vi "FINALPELLET_Jaredcopy.vi"(0 "NXT/EV3":T1) -> (1 "Material Binary":string, 2 "Type Binary":string)   [LabVIEW 2016]
uses:
  <vilib>/NXT/Subs/LVHSConnector.ctl
  <vilib>/NXT/LegoClasses/BrickReference/BrickReference.lvclass
  <vilib>/NXT/Block Support/NXT_InputPort.ctl
  <vilib>/NXT/Block Support/NXT_OutputPort.ctl
  <vilib>/NXT/Dual Mode Library/Sensors/EV3_Color_Color.vi
  <vilib>/NXT/NXTIO Xnodes/NXTIONodeSubVIs/NXTMotorRunDistance.vi
  <vilib>/NXT/Dual Mode Library/Waits/Wait_Num.vi
  <vilib>/NXT/NXTIO Xnodes/NXTIONodeSubVIs/NXTStopMotors.vi
  <vilib>/NXT/Dual Mode Library/Sensors/EV3_Color_RGB.vi
  <vilib>/NXT/NXTIO Xnodes/AddressXNode/NXTIOAddress.xnode
  <vilib>/NXT/NXTIO Xnodes/NXTIOXNode/NXTIO.xnode
panel:
  out "Material":dbl[](array[numeric])
  out "Type":dbl[](array[numeric])
  in  "Time 2":dbl
  in  "Pause":dbl
  in  "Time 1":dbl
  out "Type":string[](array[string])
  out "Type Binary":string[](array[string])
  out "Material":string[](array[string])
  out "Material Binary":string[](array[string])
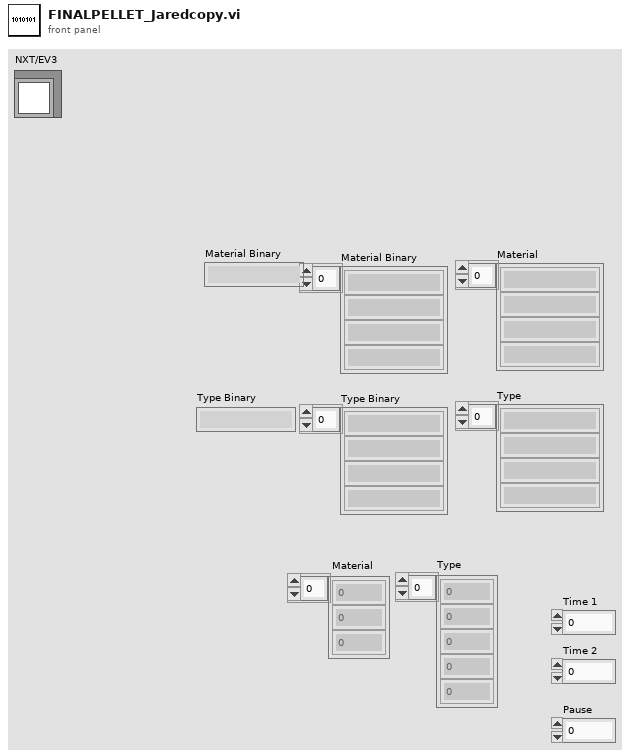
[diagram p1: front panel]
types:
  T1 = typedef "LVHSConnector.ctl" = refnum<class "BrickReference.lvclass">
  T2 = typedef "NXT_InputPort.ctl" = u32
  T3 = typedef "ColorSensorColors.ctl" = enum16{"No Color", "Black", "Blue", "Green", "Yellow", "Red", "White", "Brown"}
  T4 = typedef "NXT_OutputPort.ctl" = u8
  T5 = cluster{"[0]":string, "[1]":string, "[2]":string, "[3]":string, "[4]":string, "[5]":string, "[6]":string, "[7]":string, "[8]":string}
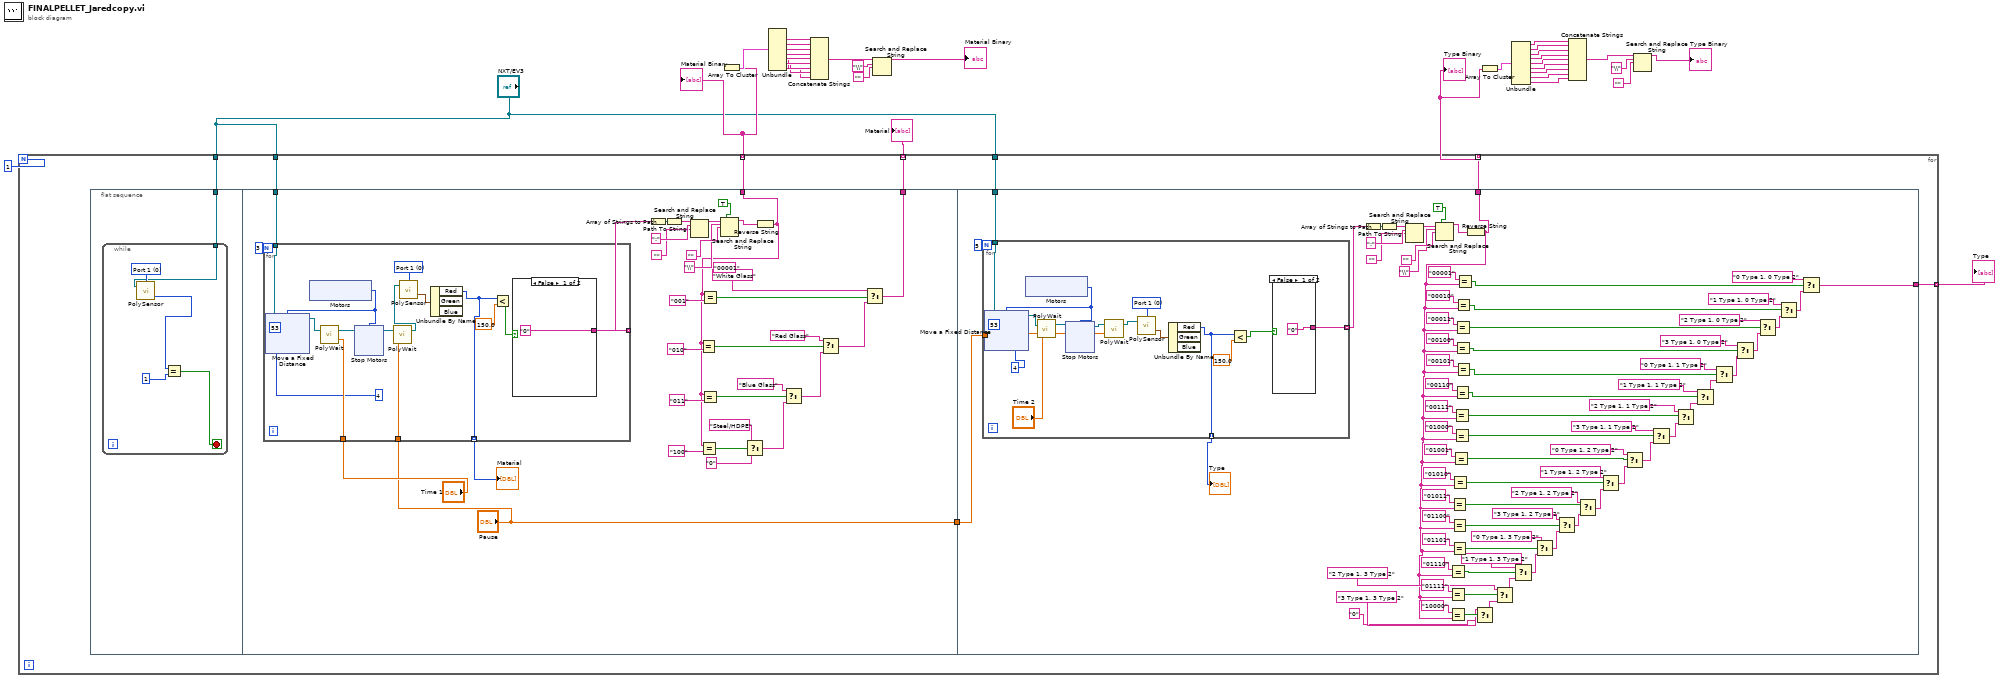
[diagram p0: block diagram]
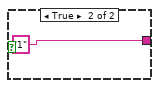
[diagram p2: hidden frame]
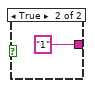
[diagram p3: hidden frame]
diagram:
  n1 = for {
    N: 1 -> [_]
    tunnel: [w42] -> w33 mode=indexing
    tunnel: [w41] -> w32 mode=indexing
    tunnel: [w40] -> w31 mode=indexing
    tunnel: [w39] -> w10 mode=indexing
    tunnel: "NXT/EV3" -> [w37]
    tunnel: "NXT/EV3" -> [w36]
    tunnel: "NXT/EV3" -> [w35]
    n2 = flat-sequence {
      tunnel: w37 -> [w43]
      tunnel: [w66] -> w42
      tunnel: [w52] -> w39
      tunnel: ["Pause"] -> w38
      tunnel: w36 -> [w49]
      tunnel: [w129] -> w41
      tunnel: [w117] -> w40
      tunnel: w38 -> [w121]
      tunnel: w35 -> [w116]
      frame #0 {
        n3 = while {
          tunnel: w43 -> [w44]
          stop <- w46 stop-if-true
          w45 = T2 0 items=["Port 1", "Port 2", "Port 3", "Port 4"] ("Port (Port 1)")
          n4 = call-poly <vilib>:"PolySensor.vi"("NXT/EV3"=w44, "Port (Port 1)"=w45) -> ("Detected Color"=w48:T3)  [unwired: 1 in, 1 out]
          n5 = Equal?(x=w48, y=1) -> (x = y?=w46:bool)
        }
      }
      frame #1 {
        (unwired) "00001"
        n6 = for {
          N: 3 -> [_]
          tunnel: [w97] -> w54 mode=indexing
          tunnel: "Time 1" -> [w95]
          tunnel: "Pause" -> [w93]
          tunnel: [w88] -> w55 mode=indexing
          tunnel: w49 -> [w82]
          w92 = T2 0 items=["Port 1", "Port 2", "Port 3", "Port 4"] ("Port (Port 1)")
          n7 = xnode "Motors"() -> ("Motor"=w84:T4)
          n8 = xnode "Move a Fixed Distance"("Speed 1"=4, "Distance 1"=53, "Motors"=w84, "NXT/EV3"=w82) -> ("NXT/EV3"=w85:T1)
          n9 = call-poly <vilib>:"PolyWait.vi"("Time (1 sec)"=w95, "NXT/EV3"=w85) -> ("NXT/EV3"=w96:T1)  [unwired: 2 in]
          n10 = xnode "Stop Motors"("Motors"=w84, "NXT/EV3"=w96) -> ("NXT/EV3"=w94:T1)
          n11 = call-poly <vilib>:"PolyWait.vi"("Time (1 sec)"=w93, "NXT/EV3"=w94) -> ("NXT/EV3"=w89:T1)  [unwired: 2 in]
          n12 = call-poly <vilib>:"PolySensor.vi"("NXT/EV3"=w89, "Port (Port 1)"=w92) -> ("RGB Color"=w87:cluster{"Red":u8, "Green":u8, "Blue":u8})  [unwired: 1 in, 1 out]
          n13 = Unbundle By Name(w87) -> ("Red"=w88:u8)  [unwired: 2 out]
          n14 = Less?(x=w88, y=150.0) -> (x < y?=w90:bool)
          n15 = case shown="False" w90 {
            tunnel: ["0" "1"] -> w97
            frame False {
            }
            frame True {
            }
          }
        }
        "Material" <- w55
        n16 = Array of Strings to Path(0:w54) -> (2:w65:path)  [unwired: 1 in]
        n17 = Path To String(path=w65) -> (string=w64:string)
        n18 = Search and Replace String(input string=w64, search string=":", replace string="") -> (result string=w61:string)  [unwired: 5 in, 3 out]
        n19 = Search and Replace String(replace all?=TRUE, input string=w61, search string="\\", replace string="") -> (result string=w53:string)  [unwired: 4 in, 3 out]
        n20 = Reverse String(1:w53) -> (0:w52:string)
        n21 = Equal?(x=w52, y="010") -> (x = y?=w51:bool)
        n22 = Equal?(x=w52, y="100") -> (x = y?=w70:bool)
        n23 = Equal?(x=w52, y="011") -> (x = y?=w71:bool)
        n24 = Equal?(x=w52, y="001") -> (x = y?=w50:bool)
        n25 = Select(t="Steel/HDPE", s=w70, f="0") -> (s? t:f=w69:string)
        n26 = Select(t="Blue Glass", s=w71, f=w69) -> (s? t:f=w73:string)
        n27 = Select(t="Red Glass", s=w51, f=w73) -> (s? t:f=w75:string)
        n28 = Select(t="White Glass", s=w50, f=w75) -> (s? t:f=w66:string)
      }
      frame #2 {
        n29 = for {
          N: 5 -> [_]
          tunnel: [w210] -> w119 mode=indexing
          tunnel: w121 -> [w208]
          tunnel: [w201] -> w120 mode=indexing
          tunnel: w116 -> [w196]
          w211 = T2 0 items=["Port 1", "Port 2", "Port 3", "Port 4"] ("Port (Port 1)")
          n30 = xnode "Motors"() -> ("Motor"=w198:T4)
          n31 = xnode "Move a Fixed Distance"("Speed 1"=4, "Distance 1"=53, "Motors"=w198, "NXT/EV3"=w196) -> ("NXT/EV3"=w199:T1)
          n32 = call-poly <vilib>:"PolyWait.vi"("Time (1 sec)"="Time 2", "NXT/EV3"=w199) -> ("NXT/EV3"=w209:T1)  [unwired: 2 in]
          n33 = xnode "Stop Motors"("Motors"=w198, "NXT/EV3"=w209) -> ("NXT/EV3"=w207:T1)
          n34 = call-poly <vilib>:"PolyWait.vi"("Time (1 sec)"=w208, "NXT/EV3"=w207) -> ("NXT/EV3"=w206:T1)  [unwired: 2 in]
          n35 = call-poly <vilib>:"PolySensor.vi"("NXT/EV3"=w206, "Port (Port 1)"=w211) -> ("RGB Color"=w204:cluster{"Red":u8, "Green":u8, "Blue":u8})  [unwired: 1 in, 1 out]
          n36 = Unbundle By Name(w204) -> ("Red"=w201:u8)  [unwired: 2 out]
          n37 = Less?(x=w201, y=150.0) -> (x < y?=w202:bool)
          n38 = case shown="False" w202 {
            tunnel: ["0" "1"] -> w210
            frame False {
            }
            frame True {
            }
          }
        }
        "Type" <- w120
        n39 = Array of Strings to Path(0:w119) -> (2:w194:path)  [unwired: 1 in]
        n40 = Path To String(path=w194) -> (string=w128:string)
        n41 = Search and Replace String(input string=w128, search string=":", replace string="") -> (result string=w125:string)  [unwired: 5 in, 3 out]
        n42 = Search and Replace String(replace all?=TRUE, input string=w125, search string="\\", replace string="") -> (result string=w118:string)  [unwired: 4 in, 3 out]
        n43 = Reverse String(1:w118) -> (0:w117:string)
        n44 = Equal?(x="01111", y=w117) -> (x = y?=w176:bool)
        n45 = Equal?(x="10000", y=w117) -> (x = y?=w177:bool)
        n46 = Equal?(x="01110", y=w117) -> (x = y?=w175:bool)
        n47 = Equal?(x="01011", y=w117) -> (x = y?=w172:bool)
        n48 = Equal?(x="01100", y=w117) -> (x = y?=w173:bool)
        n49 = Equal?(x="01101", y=w117) -> (x = y?=w174:bool)
        n50 = Equal?(x="01010", y=w117) -> (x = y?=w171:bool)
        n51 = Equal?(x="01001", y=w117) -> (x = y?=w170:bool)
        n52 = Equal?(x="00111", y=w117) -> (x = y?=w168:bool)
        n53 = Equal?(x="01000", y=w117) -> (x = y?=w169:bool)
        n54 = Equal?(x="00110", y=w117) -> (x = y?=w167:bool)
        n55 = Equal?(x="00011", y=w117) -> (x = y?=w164:bool)
        n56 = Equal?(x="00100", y=w117) -> (x = y?=w165:bool)
        n57 = Equal?(x="00010", y=w117) -> (x = y?=w163:bool)
        n58 = Equal?(x="00101", y=w117) -> (x = y?=w166:bool)
        n59 = Equal?(x="00001", y=w117) -> (x = y?=w162:bool)
        n60 = Select(t="3 Type 1, 3 Type 2", s=w177, f="0") -> (s? t:f=w161:string)
        n61 = Select(t="2 Type 1, 3 Type 2", s=w176, f=w161) -> (s? t:f=w160:string)
        n62 = Select(t="1 Type 1, 3 Type 2", s=w175, f=w160) -> (s? t:f=w159:string)
        n63 = Select(t="0 Type 1, 3 Type 2", s=w174, f=w159) -> (s? t:f=w158:string)
        n64 = Select(t="3 Type 1, 2 Type 2", s=w173, f=w158) -> (s? t:f=w157:string)
        n65 = Select(t="2 Type 1, 2 Type 2", s=w172, f=w157) -> (s? t:f=w156:string)
        n66 = Select(t="1 Type 1, 2 Type 2", s=w171, f=w156) -> (s? t:f=w155:string)
        n67 = Select(t="0 Type 1, 2 Type 2", s=w170, f=w155) -> (s? t:f=w154:string)
        n68 = Select(t="3 Type 1, 1 Type 2", s=w169, f=w154) -> (s? t:f=w153:string)
        n69 = Select(t="2 Type 1, 1 Type 2", s=w168, f=w153) -> (s? t:f=w152:string)
        n70 = Select(t="1 Type 1, 1 Type 2", s=w167, f=w152) -> (s? t:f=w151:string)
        n71 = Select(t="0 Type 1, 1 Type 2", s=w166, f=w151) -> (s? t:f=w150:string)
        n72 = Select(t="3 Type 1, 0 Type 2", s=w165, f=w150) -> (s? t:f=w149:string)
        n73 = Select(t="2 Type 1, 0 Type 2", s=w164, f=w149) -> (s? t:f=w148:string)
        n74 = Select(t="1 Type 1, 0 Type 2", s=w163, f=w148) -> (s? t:f=w147:string)
        n75 = Select(t="0 Type 1, 0 Type 2", s=w162, f=w147) -> (s? t:f=w129:string)
      }
    }
  }
  "Material Binary" <- w10
  "Material" <- w33
  "Type" <- w32
  "Type Binary" <- w31
  n76 = Array To Cluster(array=w10) -> (cluster=w20:T5)
  n77 = Unbundle(w20) -> ("[0]"=w19:string, "[1]"=w18:string, "[2]"=w17:string, "[3]"=w16:string, "[4]"=w15:string, "[5]"=w14:string, "[6]"=w13:string, "[7]"=w12:string, "[8]"=w11:string)
  n78 = Concatenate Strings(w19, w18, w17, w16, w15, w14, w13, w12, w11) -> (w8:string)
  n79 = Search and Replace String(input string=w8, search string="\\", replace string="") -> (result string=→"Material Binary":string)  [unwired: 5 in, 3 out]
  n80 = Array To Cluster(array=w31) -> (cluster=w30:T5)
  n81 = Unbundle(w30) -> ("[0]"=w29:string, "[1]"=w28:string, "[2]"=w27:string, "[3]"=w26:string, "[4]"=w25:string, "[5]"=w24:string, "[6]"=w23:string, "[7]"=w22:string, "[8]"=w21:string)
  n82 = Concatenate Strings(w29, w28, w27, w26, w25, w24, w23, w22, w21) -> (w2:string)
  n83 = Search and Replace String(input string=w2, search string="\\", replace string="") -> (result string=→"Type Binary":string)  [unwired: 5 in, 3 out]
